vi "TEST - Delete Elements from 2D Array.vi"(8 "error in (no error)":errorcluster) -> (0 "error out":errorcluster, 2 "Pass?":bool=TRUE)   [LabVIEW 2020]
doc: "This VI template can be used for the functional testing of VIs; this implementation includes handling for the testing of polymorphic VIs, and the polymorphic elements should be removed if not needed.\n\nCoded by Douglas A. Femec, January 24, 2006.\n\nCopyright (c) 2005-2006 MKS Instruments, Inc.\nAll rights reserved."
uses:
  TEST - Delete Elements from 2D Array - Inputs.ctl
  Polymorphizer+ Data Type.ctl
  TEST - Delete Elements from 2D Array - Outputs.ctl
  source/library/Delete Elements from Array/Delete Elements from 2D Array (EXT).vi
  source/library/Delete Elements from Array/Delete Elements from 2D Array (I64).vi
  source/library/Delete Elements from Array/Delete Elements from 2D Array (U64).vi
  source/library/Delete Elements from Array/Delete Elements from 2D Array (DBL).vi
  source/library/Delete Elements from Array/Delete Elements from 2D Array (SGL).vi
  source/library/Delete Elements from Array/Delete Elements from 2D Array (I32).vi
  source/library/Delete Elements from Array/Delete Elements from 2D Array (I16).vi
  source/library/Delete Elements from Array/Delete Elements from 2D Array (I8).vi
  source/library/Delete Elements from Array/Delete Elements from 2D Array (LVObject).vi
  source/library/Delete Elements from Array/Delete Elements from 2D Array (U32).vi
  source/library/Delete Elements from Array/Delete Elements from 2D Array (U16).vi
  source/library/Delete Elements from Array/Delete Elements from 2D Array (U8).vi
  source/library/Delete Elements from Array/Delete Elements from 2D Array (CXT).vi
  source/library/Delete Elements from Array/Delete Elements from 2D Array (CDB).vi
  source/library/Delete Elements from Array/Delete Elements from 2D Array (CSG).vi
  source/library/Delete Elements from Array/Delete Elements from 2D Array (Boolean).vi
  source/library/Delete Elements from Array/Delete Elements from 2D Array (String).vi
  source/library/Delete Elements from Array/Delete Elements from 2D Array (Path).vi
  source/library/Delete Elements from Array/Delete Elements from 2D Array (Variant).vi
  source/library/openg_array.lvlib
  TestClass/TestClass.lvclass
panel:
  out "Pass Array":bool[][](array[boolean])
  out "Generated Outputs":T1[][](array[typedef])=[[{"Description"="expect empty array", "array w/ subset deleted"=[], "deleted elements"=[]}, {"Description"="expect empty array", "array w/ subset deleted"=[], "deleted elements"=[]}, {"Description"="expect empty array", "array w/ subset deleted"=[], "deleted elements"=[]}, {"Description"="expect empty array", "array w/ subset deleted"=[], "deleted elements"=[]}, {"Description"="expect empty array", "array w/ subset deleted"=[], "deleted elements"=[]}, {"Description"="expect empty array", "array w/ subset deleted"=[], "deleted elements"=[]}, {"Description"="expect empty array", "array w/ subset deleted"=[], "deleted elements"=[]}, {"Description"="expect empty array", "array w/ subset deleted"=[], "deleted elements"=[]}, {"Description"="expect empty array", "array w/ subset deleted"=[], "deleted elements"=[]}, {"Description"="expect empty array", "array w/ subset deleted"=[], "deleted elements"=[]}, {"Description"="expect empty array", "array w/ subset deleted"=[], "deleted elements"=[]}, {"Description"="expect empty array", "array w/ subset deleted"=[], "deleted elements"=[]}, {"Description"="expect empty array", "array w/ subset deleted"=[], "deleted elements"=[]}, {"Description"="expect empty array", "array w/ subset deleted"=[], "deleted elements"=[]}, {"Description"="expect empty array", "array w/ subset deleted"=[], "deleted elements"=[]}, {"Description"="expect empty array", "array w/ subset deleted"=[], "deleted elements"=[]}], [{"Description"="Some rows deleted", "array w/ subset deleted"=[[3.0, 4.0], [7.0, 8.0]], "deleted elements"=[[5.0, 6.0], [1.0, 2.0]]}, {"Description"="Some rows deleted", "array w/ subset deleted"=[[3.0, 4.0], [7.0, 8.0]], "deleted elements"=[[5.0, 6.0], [1.0, 2.0]]}, {"Description"="Some rows deleted", "array w/ subset deleted"=[[3.0, 4.0], [7.0, 8.0]], "deleted elements"=[[5.0, 6.0], [1.0, 2.0]]}, {"Description"="Some rows deleted", "array w/ subset deleted"=[[3.0, 4.0], [7.0, 8.0]], "deleted elements"=[[5.0, 6.0], [1.0, 2.0]]}, {"Description"="Some rows deleted", "array w/ subset deleted"=[[3.0, 4.0], [7.0, 8.0]], "deleted elements"=[[5.0, 6.0], [1.0, 2.0]]}, {"Description"="Some rows deleted", "array w/ subset deleted"=[[3.0, 4.0], [7.0, 8.0]], "deleted elements"=[[5.0, 6.0], [1.0, 2.0]]}, {"Description"="Some rows deleted", "array w/ subset deleted"=[[3.0, 4.0], [7.0, 8.0]], "deleted elements"=[[5.0, 6.0], [1.0, 2.0]]}, {"Description"="Some rows deleted", "array w/ subset deleted"=[[3.0, 4.0], [7.0, 8.0]], "deleted elements"=[[5.0, 6.0], [1.0, 2.0]]}, {"Description"="Some rows deleted", "array w/ subset deleted"=[[3.0, 4.0], [7.0, 8.0]], "deleted elements"=[[5.0, 6.0], [1.0, 2.0]]}, {"Description"="Some rows deleted", "array w/ subset deleted"=[[3.0, 4.0], [7.0, 8.0]], "deleted elements"=[[5.0, 6.0], [1.0, 2.0]]}, {"Description"="Some rows deleted", "array w/ subset deleted"=[[3.0, 4.0], [7.0, 8.0]], "deleted elements"=[[5.0, 6.0], [1.0, 2.0]]}, {"Description"="Some rows deleted", "array w/ subset deleted"=[[3.0, 4.0], [7.0, 8.0]], "deleted elements"=[[5.0, 6.0], [1.0, 2.0]]}, {"Description"="Some rows deleted", "array w/ subset deleted"=[[3.0, 4.0], [7.0, 8.0]], "deleted elements"=[[5.0, 6.0], [1.0, 2.0]]}, {"Description"="Some rows deleted", "array w/ subset deleted"=[[3.0, 4.0], [7.0, 8.0]], "deleted elements"=[[5.0, 6.0], [1.0, 2.0]]}, {"Description"="Some rows deleted", "array w/ subset deleted"=[[3.0, 4.0], [7.0, 8.0]], "deleted elements"=[[5.0, 6.0], [1.0, 2.0]]}, {"Description"="", "array w/ subset deleted"=[], "deleted elements"=[]}], [{"Description"="", "array w/ subset deleted"=[], "deleted elements"=[]}, {"Description"="", "array w/ subset deleted"=[], "deleted elements"=[]}, {"Description"="", "array w/ subset deleted"=[], "deleted elements"=[]}, {"Description"="", "array w/ subset deleted"=[], "deleted elements"=[]}, {"Description"="", "array w/ subset deleted"=[], "deleted elements"=[]}, {"Description"="", "array w/ subset deleted"=[], "deleted elements"=[]}, {"Description"="", "array w/ subset deleted"=[], "deleted elements"=[]}, {"Description"="", "array w/ subset deleted"=[], "deleted elements"=[]}, {"Description"="", "array w/ subset deleted"=[], "deleted elements"=[]}, {"Description"="", "array w/ subset deleted"=[], "deleted elements"=[]}, {"Description"="", "array w/ subset deleted"=[], "deleted elements"=[]}, {"Description"="", "array w/ subset deleted"=[], "deleted elements"=[]}, {"Description"="", "array w/ subset deleted"=[], "deleted elements"=[]}, {"Description"="", "array w/ subset deleted"=[], "deleted elements"=[]}, {"Description"="", "array w/ subset deleted"=[], "deleted elements"=[]}, {"Description"="", "array w/ subset deleted"=[], "deleted elements"=[]}], [{"Description"="", "array w/ subset deleted"=[], "deleted elements"=[]}, {"Description"="", "array w/ subset deleted"=[], "deleted elements"=[]}, {"Description"="", "array w/ subset deleted"=[], "deleted elements"=[]}, {"Description"="", "array w/ subset deleted"=[], "deleted elements"=[]}, {"Description"="", "array w/ subset deleted"=[], "deleted elements"=[]}, {"Description"="", "array w/ subset deleted"=[], "deleted elements"=[]}, {"Description"="", "array w/ subset deleted"=[], "deleted elements"=[]}, {"Description"="", "array w/ subset deleted"=[], "deleted elements"=[]}, {"Description"="", "array w/ subset deleted"=[], "deleted elements"=[]}, {"Description"="", "array w/ subset deleted"=[], "deleted elements"=[]}, {"Description"="", "array w/ subset deleted"=[], "deleted elements"=[]}, {"Description"="", "array w/ subset deleted"=[], "deleted elements"=[]}, {"Description"="", "array w/ subset deleted"=[], "deleted elements"=[]}, {"Description"="", "array w/ subset deleted"=[], "deleted elements"=[]}, {"Description"="", "array w/ subset deleted"=[], "deleted elements"=[]}, {"Description"="", "array w/ subset deleted"=[], "deleted elements"=[]}]] {"deleted elements" format="%.2f"; "array w/ subset deleted" format="%.2f"}
  in  "Expected Outputs":T1[](array[typedef])=[{"Description"="expect empty array", "array w/ subset deleted"=[], "deleted elements"=[]}, {"Description"="Some rows deleted", "array w/ subset deleted"=[[3.0, 4.0, 10.0], [7.0, 8.0, 12.0]], "deleted elements"=[[5.0, 6.0, 11.0], [1.0, 2.0, 9.0]]}, {"Description"="Some columns deleted", "array w/ subset deleted"=[[2.0, 4.0], [6.0, 8.0], [10.0, 12.0]], "deleted elements"=[[3.0, 1.0], [7.0, 5.0], [11.0, 9.0]]}, {"Description"="", "array w/ subset deleted"=[], "deleted elements"=[]}] {"deleted elements" format="%.2f"; "array w/ subset deleted" format="%.2f"}
  in  "Inputs":T2[](array[typedef])=[{"Description"="Empty array", "Data Types to Test"=[enum."EXT", enum."DBL", enum."SGL", enum."I32", enum."I16", enum."I8", enum."U32", enum."U16", enum."U8", enum."CXT", enum."CDB", enum."CSG", enum."Boolean", enum."String", enum."Path", enum."Variant", enum."I64", enum."U64", enum."LabVIEW Object"], "Array"=[], "Indices"=[], "delete (rows or columns)"=enum."rows"}, {"Description"="Delete some rows", "Data Types to Test"=[enum."EXT", enum."DBL", enum."SGL", enum."I32", enum."I16", enum."I8", enum."U32", enum."U16", enum."U8", enum."CXT", enum."CDB", enum."CSG", enum."Boolean", enum."String", enum."Path", enum."Variant", enum."I64", enum."U64", enum."LabVIEW Object"], "Array"=[[1.0, 2.0, 9.0], [3.0, 4.0, 10.0], [5.0, 6.0, 11.0], [7.0, 8.0, 12.0]], "Indices"=[2, 0], "delete (rows or columns)"=enum."rows"}, {"Description"="Delete some columns", "Data Types to Test"=[enum."EXT", enum."DBL", enum."SGL", enum."I32", enum."I16", enum."I8", enum."U32", enum."U16", enum."U8", enum."CXT", enum."CDB", enum."CSG", enum."Boolean", enum."String", enum."Path", enum."Variant", enum."I64", enum."U64", enum."LabVIEW Object"], "Array"=[[1.0, 2.0, 3.0, 4.0], [5.0, 6.0, 7.0, 8.0], [9.0, 10.0, 11.0, 12.0]], "Indices"=[2, 0], "delete (rows or columns)"=enum."columns"}, {"Description"="", "Data Types to Test"=[enum."EXT", enum."DBL", enum."SGL", enum."I32", enum."I16", enum."I8", enum."U32", enum."U16", enum."U8", enum."CXT", enum."CDB", enum."CSG", enum."Boolean", enum."String", enum."Path", enum."Variant", enum."I64", enum."U64", enum."LabVIEW Object"], "Array"=[], "Indices"=[], "delete (rows or columns)"=enum."rows"}] {"Array" format="%.2f"}
  # "Copyright (c) 2005-2006 MKS Instruments, Inc.\nAll rights reserved."
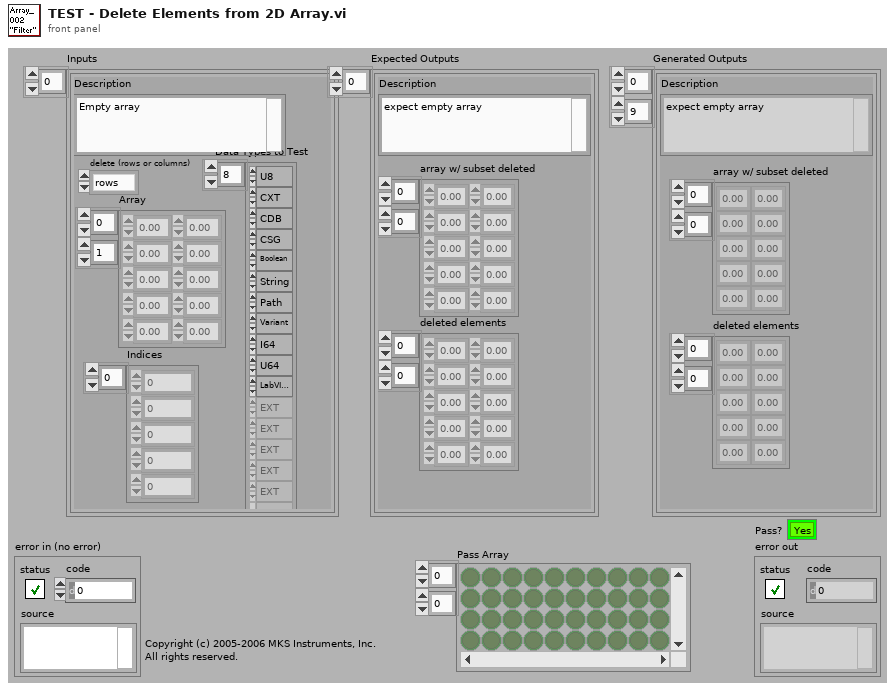
[diagram p1: front panel]
types:
  T1 = typedef "TEST - Delete Elements from 2D Array - Outputs.ctl" = cluster{"Description":string, "array w/ subset deleted":sgl[][], "deleted elements":sgl[][]}
  T2 = typedef "TEST - Delete Elements from 2D Array - Inputs.ctl" = cluster{"Description":string, "Data Types to Test":T3[], "Array":sgl[][], "Indices":i32[], "delete (rows or columns)":enum16{"rows", "columns"}}
  T3 = typedef "Polymorphizer+ Data Type.ctl" = enum16{"EXT", "DBL", "SGL", "I32", "I16", "I8", "U32", "U16", "U8", "CXT", "CDB", "CSG", "Boolean", "String", "Path", "Variant", "CTL-REF", "GEN-REF", "GObj-REF", "VI-REF", "ENUM", "ERR", "FILE-REF", "MENU-REF", "MENU-RING", "PICT-RING", "TXT&PICT-RING", "TXT-RING", "I64", "U64", "LabVIEW Object"}
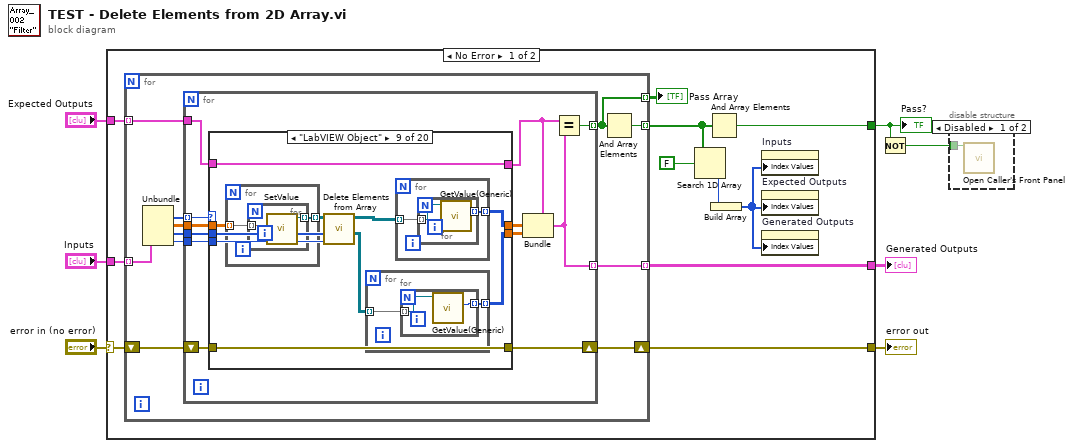
[diagram p0: block diagram]
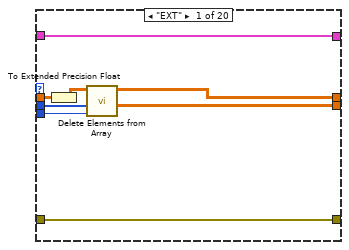
[diagram p3: hidden frame]
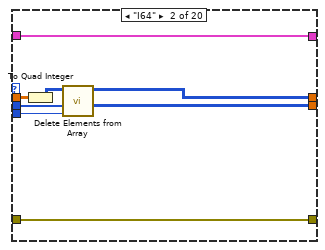
[diagram p4: hidden frame]
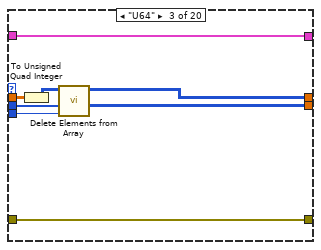
[diagram p5: hidden frame]
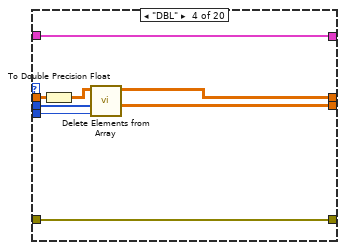
[diagram p6: hidden frame]
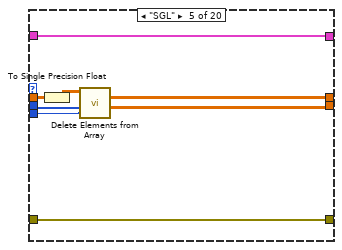
[diagram p7: hidden frame]
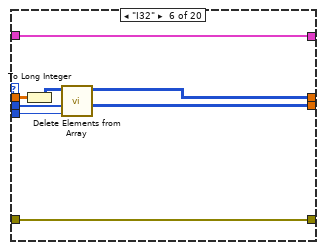
[diagram p8: hidden frame]
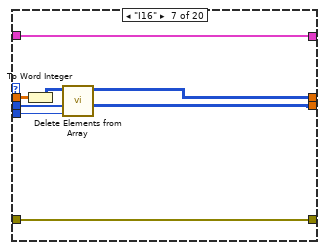
[diagram p9: hidden frame]
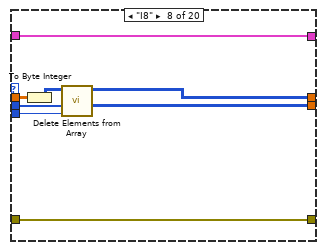
[diagram p10: hidden frame]
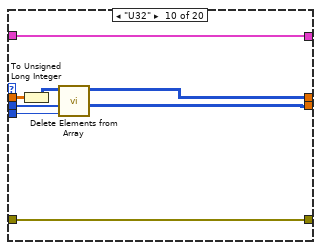
[diagram p11: hidden frame]
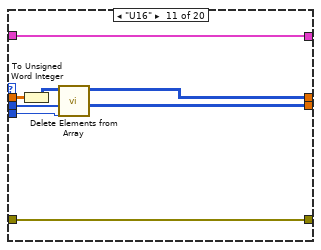
[diagram p12: hidden frame]
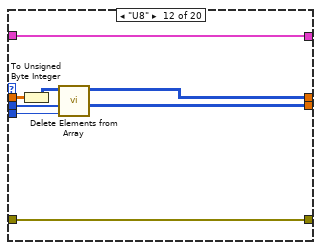
[diagram p13: hidden frame]
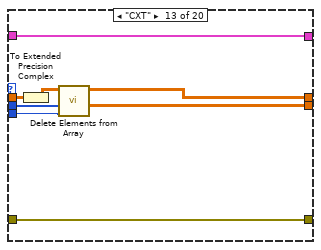
[diagram p14: hidden frame]
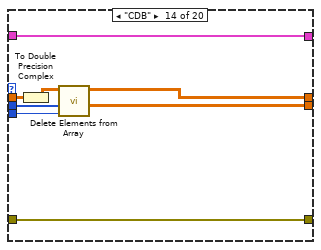
[diagram p15: hidden frame]
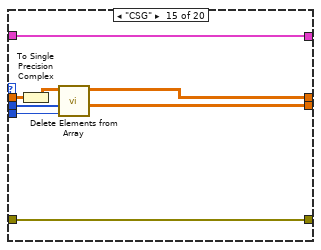
[diagram p16: hidden frame]
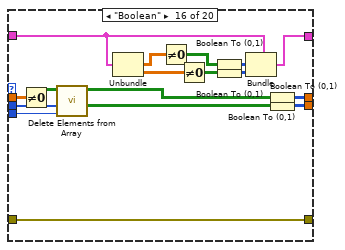
[diagram p17: hidden frame]
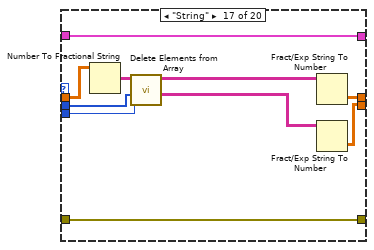
[diagram p18: hidden frame]
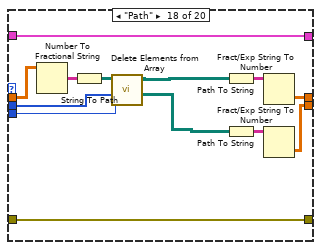
[diagram p19: hidden frame]
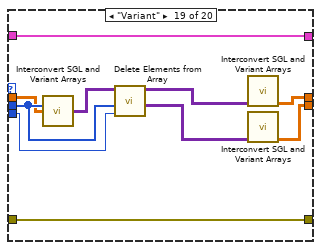
[diagram p20: hidden frame]
diagram:
  n1 = case shown="No Error" "error in (no error)" {
    selector: "error in (no error)" -> [w17 w230]
    tunnel: [w18 w230] -> w6
    tunnel: "Expected Outputs" -> [w15 _]
    tunnel: "Inputs" -> [w16 _]
    tunnel: [w14 _] -> w3
    tunnel: [w13 _] -> w2
    frame No Error {
      n2 = for {
        shift-right: [w25] -> w18
        shift-left: w17 -> [w26]
        tunnel: w16 -> [w27] mode=indexing
        tunnel: w15 -> [w29] mode=indexing
        tunnel: [w28] -> w14 mode=indexing
        tunnel: [w24] -> w12 mode=indexing
        tunnel: [w19] -> w8 mode=indexing
        n3 = Unbundle(w27) -> ("Data Types to Test"=w23:T3[], "Array"=w21:sgl[][], "Indices"=w22:i32[], "delete (rows or columns)"=w20:enum16{"rows", "columns"})  [unwired: 1 out]
        n4 = for {
          tunnel: w29 -> [w32]
          tunnel: [w30] -> w28 mode=indexing
          tunnel: [w41] -> w19 mode=indexing
          shift-right: [w36] -> w25
          shift-left: w26 -> [w37]
          tunnel: w23 -> [w38] mode=indexing
          tunnel: w21 -> [w40]
          tunnel: w22 -> [w39]
          tunnel: w20 -> [w33]
          n5 = case shown="\"LabVIEW Object\"" w38 {
            tunnel: w40 -> [w49 w57 w65 w73 w81 w89 w97 w105 w112 w135 w143 w151 w159 w167 w175 w192 w202 w214 w223 w228]
            tunnel: [w45 w53 w61 w69 w77 w85 w92 w100 w109 w130 w138 w146 w154 w162 w170 w191 w201 w213 w218 w228] -> w35
            tunnel: w39 -> [w46 w54 w62 w71 w78 w87 w95 w103 w114 w133 w141 w149 w157 w165 w173 w188 w199 w210 w224 _]
            tunnel: w37 -> [w48 w56 w64 w72 w80 w88 w96 w104 w115 w134 w142 w150 w158 w166 w174 w190 w200 w211 w225 w229]
            tunnel: [w48 w56 w64 w72 w80 w88 w96 w104 w115 w134 w142 w150 w158 w166 w174 w190 w200 w211 w225 w229] -> w36
            tunnel: [w44 w52 w60 w68 w76 w84 w93 w101 w107 w131 w139 w147 w155 w163 w171 w186 w195 w205 w219 cxt[][] []] -> w34
            tunnel: w33 -> [w43 w51 w59 w67 w75 w83 w91 w99 w113 w129 w137 w145 w153 w161 w169 w184 w194 w204 w217 _]
            tunnel: [w42 w50 w58 w66 w74 w82 w90 w98 w106 w128 w136 w144 w152 w160 w168 w183 w193 w203 w216 w226] -> w31
            tunnel: w32 -> [w42 w50 w58 w66 w74 w82 w90 w98 w106 w128 w136 w144 w152 w160 w168 w182 w193 w203 w216 w226]
            frame "EXT" {
              n6 = To Extended Precision Float(1:w49) -> (0:w47:ext[][])
              n7 = call-poly "Delete Elements from Array.vi"("delete (rows or columns)"=w43, "indices"=w46, "array"=w47) -> ("deleted elements"=w44:ext[][], "array w/ subset deleted"=w45:ext[][])  [unwired: 7 in]
            }
            frame "I64" {
              n8 = To Quad Integer(1:w57) -> (0:w55:i64[][])
              n9 = call-poly "Delete Elements from Array.vi"("delete (rows or columns)"=w51, "indices"=w54, "array"=w55) -> ("deleted elements"=w52:i64[][], "array w/ subset deleted"=w53:i64[][])  [unwired: 7 in]
            }
            frame "U64" {
              n10 = To Unsigned Quad Integer(1:w65) -> (0:w63:u64[][])
              n11 = call-poly "Delete Elements from Array.vi"("delete (rows or columns)"=w59, "indices"=w62, "array"=w63) -> ("deleted elements"=w60:u64[][], "array w/ subset deleted"=w61:u64[][])  [unwired: 7 in]
            }
            frame "DBL" {
              n12 = To Double Precision Float(number=w73) -> (double precision float=w70:dbl[][])
              n13 = call-poly "Delete Elements from Array.vi"("delete (rows or columns)"=w67, "indices"=w71, "array"=w70) -> ("deleted elements"=w68:dbl[][], "array w/ subset deleted"=w69:dbl[][])  [unwired: 7 in]
            }
            frame "SGL" {
              n14 = To Single Precision Float(number=w81) -> (single precision float=w79:sgl[][])
              n15 = call-poly "Delete Elements from Array.vi"("delete (rows or columns)"=w75, "indices"=w78, "array"=w79) -> ("deleted elements"=w76:sgl[][], "array w/ subset deleted"=w77:sgl[][])  [unwired: 7 in]
            }
            frame "I32" {
              n16 = To Long Integer(number=w89) -> (32bit integer=w86:i32[][])
              n17 = call-poly "Delete Elements from Array.vi"("delete (rows or columns)"=w83, "indices"=w87, "array"=w86) -> ("deleted elements"=w84:i32[][], "array w/ subset deleted"=w85:i32[][])  [unwired: 7 in]
            }
            frame "I16" {
              n18 = To Word Integer(number=w97) -> (16bit integer=w94:i16[][])
              n19 = call-poly "Delete Elements from Array.vi"("delete (rows or columns)"=w91, "indices"=w95, "array"=w94) -> ("deleted elements"=w93:i16[][], "array w/ subset deleted"=w92:i16[][])  [unwired: 7 in]
            }
            frame "I8" {
              n20 = To Byte Integer(number=w105) -> (8bit integer=w102:i8[][])
              n21 = call-poly "Delete Elements from Array.vi"("delete (rows or columns)"=w99, "indices"=w103, "array"=w102) -> ("deleted elements"=w101:i8[][], "array w/ subset deleted"=w100:i8[][])  [unwired: 7 in]
            }
            frame "LabVIEW Object" {
              n22 = for {
                tunnel: w112 -> [w125] mode=indexing
                tunnel: [w124] -> w111 mode=indexing
                n23 = for {
                  tunnel: w125 -> [w127] mode=indexing
                  tunnel: [w126] -> w124 mode=indexing
                  n24 = call "SetValue.vi"("Value"=w127) -> ("TestClass out"=w126:refnum<class "TestClass.lvclass">)  [unwired: 9 in, 1 out]
                }
              }
              n25 = call-poly "Delete Elements from Array.vi"("delete (rows or columns)"=w113, "indices"=w114, "array"=w111) -> ("deleted elements"=w108:refnum<class>[][], "array w/ subset deleted"=w110:refnum<class>[][])  [unwired: 7 in]
              n26 = for {
                tunnel: w108 -> [w117] mode=indexing
                tunnel: [w116] -> w107 mode=indexing
                n27 = for {
                  tunnel: w117 -> [w118] mode=indexing
                  tunnel: [w119] -> w116 mode=indexing
                  n28 = call "GetValue(Generic).vi"("TestClass in"=w118) -> ("Value"=w119:i32)  [unwired: 8 in, 2 out]
                }
              }
              n29 = for {
                tunnel: w110 -> [w121] mode=indexing
                tunnel: [w120] -> w109 mode=indexing
                n30 = for {
                  tunnel: w121 -> [w122] mode=indexing
                  tunnel: [w123] -> w120 mode=indexing
                  n31 = call "GetValue(Generic).vi"("TestClass in"=w122) -> ("Value"=w123:i32)  [unwired: 8 in, 2 out]
                }
              }
            }
            frame "U32" {
              n32 = To Unsigned Long Integer(number=w135) -> (unsigned 32bit integer=w132:u32[][])
              n33 = call-poly "Delete Elements from Array.vi"("delete (rows or columns)"=w129, "indices"=w133, "array"=w132) -> ("deleted elements"=w131:u32[][], "array w/ subset deleted"=w130:u32[][])  [unwired: 7 in]
            }
            frame "U16" {
              n34 = To Unsigned Word Integer(number=w143) -> (unsigned 16bit integer=w140:u16[][])
              n35 = call-poly "Delete Elements from Array.vi"("delete (rows or columns)"=w137, "indices"=w141, "array"=w140) -> ("deleted elements"=w139:u16[][], "array w/ subset deleted"=w138:u16[][])  [unwired: 7 in]
            }
            frame "U8" {
              n36 = To Unsigned Byte Integer(number=w151) -> (unsigned 8bit integer=w148:u8[][])
              n37 = call-poly "Delete Elements from Array.vi"("delete (rows or columns)"=w145, "indices"=w149, "array"=w148) -> ("deleted elements"=w147:u8[][], "array w/ subset deleted"=w146:u8[][])  [unwired: 7 in]
            }
            frame "CXT" {
              n38 = To Extended Precision Complex(1:w159) -> (0:w156:cxt[][])
              n39 = call-poly "Delete Elements from Array.vi"("delete (rows or columns)"=w153, "indices"=w157, "array"=w156) -> ("deleted elements"=w155:cxt[][], "array w/ subset deleted"=w154:cxt[][])  [unwired: 7 in]
            }
            frame "CDB" {
              n40 = To Double Precision Complex(1:w167) -> (0:w164:cdb[][])
              n41 = call-poly "Delete Elements from Array.vi"("delete (rows or columns)"=w161, "indices"=w165, "array"=w164) -> ("deleted elements"=w163:cdb[][], "array w/ subset deleted"=w162:cdb[][])  [unwired: 7 in]
            }
            frame "CSG" {
              n42 = To Single Precision Complex(1:w175) -> (0:w172:csg[][])
              n43 = call-poly "Delete Elements from Array.vi"("delete (rows or columns)"=w169, "indices"=w173, "array"=w172) -> ("deleted elements"=w171:csg[][], "array w/ subset deleted"=w170:csg[][])  [unwired: 7 in]
            }
            frame "Boolean" {
              n44 = Not Equal To 0?(x=w192) -> (x != 0?=w189:bool[][])
              n45 = call-poly "Delete Elements from Array.vi"("delete (rows or columns)"=w184, "indices"=w188, "array"=w189) -> ("deleted elements"=w185:bool[][], "array w/ subset deleted"=w187:bool[][])  [unwired: 7 in]
              n46 = Unbundle(w182) -> ("array w/ subset deleted"=w180:sgl[][], "deleted elements"=w181:sgl[][])  [unwired: 1 out]
              n47 = Not Equal To 0?(x=w180) -> (x != 0?=w179:bool[][])
              n48 = Not Equal To 0?(x=w181) -> (x != 0?=w176:bool[][])
              n49 = Boolean To (0,1)(Boolean=w179) -> (0, 1=w178:i16[][])
              n50 = Boolean To (0,1)(Boolean=w176) -> (0, 1=w177:i16[][])
              n51 = Bundle(cluster=w182, "array w/ subset deleted"=w178, "deleted elements"=w177) -> (w183:T1)  [unwired: 1 in]
              n52 = Boolean To (0,1)(Boolean=w187) -> (0, 1=w191:i16[][])
              n53 = Boolean To (0,1)(Boolean=w185) -> (0, 1=w186:i16[][])
            }
            frame "String" {
              n54 = Number To Fractional String(number=w202) -> (F-format string=w198:string[][])  [unwired: 3 in]
              n55 = call-poly "Delete Elements from Array.vi"("delete (rows or columns)"=w194, "indices"=w199, "array"=w198) -> ("deleted elements"=w196:string[][], "array w/ subset deleted"=w197:string[][])  [unwired: 7 in]
              n56 = Fract/Exp String To Number(string=w197) -> (number=w201:dbl[][])  [unwired: 3 in, 1 out]
              n57 = Fract/Exp String To Number(string=w196) -> (number=w195:dbl[][])  [unwired: 3 in, 1 out]
            }
            frame "Path" {
              n58 = Number To Fractional String(number=w214) -> (F-format string=w215:string[][])  [unwired: 3 in]
              n59 = String To Path(string=w215) -> (path=w209:path[][])
              n60 = call-poly "Delete Elements from Array.vi"("delete (rows or columns)"=w204, "indices"=w210, "array"=w209) -> ("deleted elements"=w206:path[][], "array w/ subset deleted"=w208:path[][])  [unwired: 7 in]
              n61 = Path To String(path=w208) -> (string=w212:string[][])
              n62 = Path To String(path=w206) -> (string=w207:string[][])
              n63 = Fract/Exp String To Number(string=w212) -> (number=w213:dbl[][])  [unwired: 3 in, 1 out]
              n64 = Fract/Exp String To Number(string=w207) -> (number=w205:dbl[][])  [unwired: 3 in, 1 out]
            }
            frame "Variant" {
              n65 = call "Interconvert SGL and Variant Arrays.vi"("SGL 1D Array 2 In"=w224, "SGL 2D Array In"=w223) -> ("Variant 2D Array Out"=w222:variant[][])  [unwired: 9 in, 4 out]
              n66 = call-poly "Delete Elements from Array.vi"("delete (rows or columns)"=w217, "indices"=w224, "array"=w222) -> ("deleted elements"=w221:variant[][], "array w/ subset deleted"=w220:variant[][])  [unwired: 7 in]
              n67 = call "Interconvert SGL and Variant Arrays.vi"("Variant 2D Array In"=w220) -> ("SGL 2D Array Out"=w218:sgl[][])  [unwired: 10 in, 4 out]
              n68 = call "Interconvert SGL and Variant Arrays.vi"("Variant 2D Array In"=w221) -> ("SGL 2D Array Out"=w219:sgl[][])  [unwired: 10 in, 4 out]
            }
            frame Default {
            }
          }
          n69 = Bundle(cluster=w31, "array w/ subset deleted"=w35, "deleted elements"=w34) -> (w30:T1)  [unwired: 1 in]
          n70 = Equal?(x=w31, y=w30) -> (x = y?=w41:bool)
        }
        n71 = And Array Elements(Boolean array=w19) -> (logical AND=w24:bool)
      }
      "Pass Array" <- w8
      n72 = Search 1D Array(1D array=w12, element=FALSE) -> (index of element=w10:i32)  [unwired: 1 in]
      n73 = And Array Elements(Boolean array=w12) -> (logical AND=w13:bool)
      n74 = Build Array(w10) -> (w9:i32[])
      n75 = property on="Inputs" class="Arr (strict)"("Index Values"=w9) -> ()  [unwired: 2 in, 2 out]
      n76 = property on="Expected Outputs" class="Arr (strict)"("Index Values"=w9) -> ()  [unwired: 2 in, 2 out]
      n77 = property on="Generated Outputs" class="Arr (strict)"("Index Values"=w9) -> ()  [unwired: 2 in, 2 out]
    }
    frame Error {
    }
  }
  "error out" <- w6
  "Pass?" <- w2
  "Generated Outputs" <- w3
  n78 = Not(x=w2) -> (.not. x?=w1:bool)
  n79 = disable-structure shown="Disabled" {
    disable-tunnel: w1 -> [w231 _]
    frame Disabled {
      n80 = call "Open Caller's Front Panel.vi"("Open?"=w231) -> ()  [unwired: 14 in, 1 out]
    }
    frame Enabled {
    }
  }
